vi "RSLT_VALUE.vi"(0 "MAX-MIN Temp":cluster{"MIN":dbl, "MAX":dbl, "ACTUAL":dbl}, 3 "INPUT cluster":T2, 5 "MAX-MIN PRESSURE":cluster{"MIN":dbl, "MAX":dbl, "ACTUALLY":dbl}, 7 "MAX-MIN FLOW":cluster{"MIN":dbl, "MAX":dbl, "ACTUALLY":dbl}, 9 "CLUSTER":T3={"Files"=[], "Browse File"=path "", "TIMEOUT"=100, "GRAPH"=[{array[68443 elements], array[68443 elements]}, {array[68363 elements], array[68363 elements]}, {array[40500 elements], array[40500 elements]}], "CHL 1"={"chl1 MIN"=110.0, "chl1 MAX"=130.0, "chl1 thrshold"=120.0}, "CHL 2"={"chl2 MIN"=33.0, "chl2 MAX"=35.0, "chl2 thrshold"=25.0}, "CHL 3"={"chl3 MIN"=20.0, "chl3 MAX"=30.0, "chl3 thrshold"=34.0}, "Report File"=path "", "Data_to_report"={"date/time string"="", "User Name"="", "BARCODE"="", "SELECTED RECIPE"="", "Rst"="", "Error Code"="", "RESULT ARRAY"=[]}, "BMP"={"chl3 MIN"=0.0, "chl3 MAX"=0.0, "chl3 thrshold"=0.0}}, 11 "error in":errorcluster, 12 "ACTUAL BPM":dbl=32134659.0 format="%#_13g") -> (4 "CLUSTER TO SQL":T1, 6 "RESULT ARRAY":string[](array[string]), 15 "error OUT":errorcluster)   [LabVIEW 2017]
panel:
  out "appended array":dbl[](array[numeric])
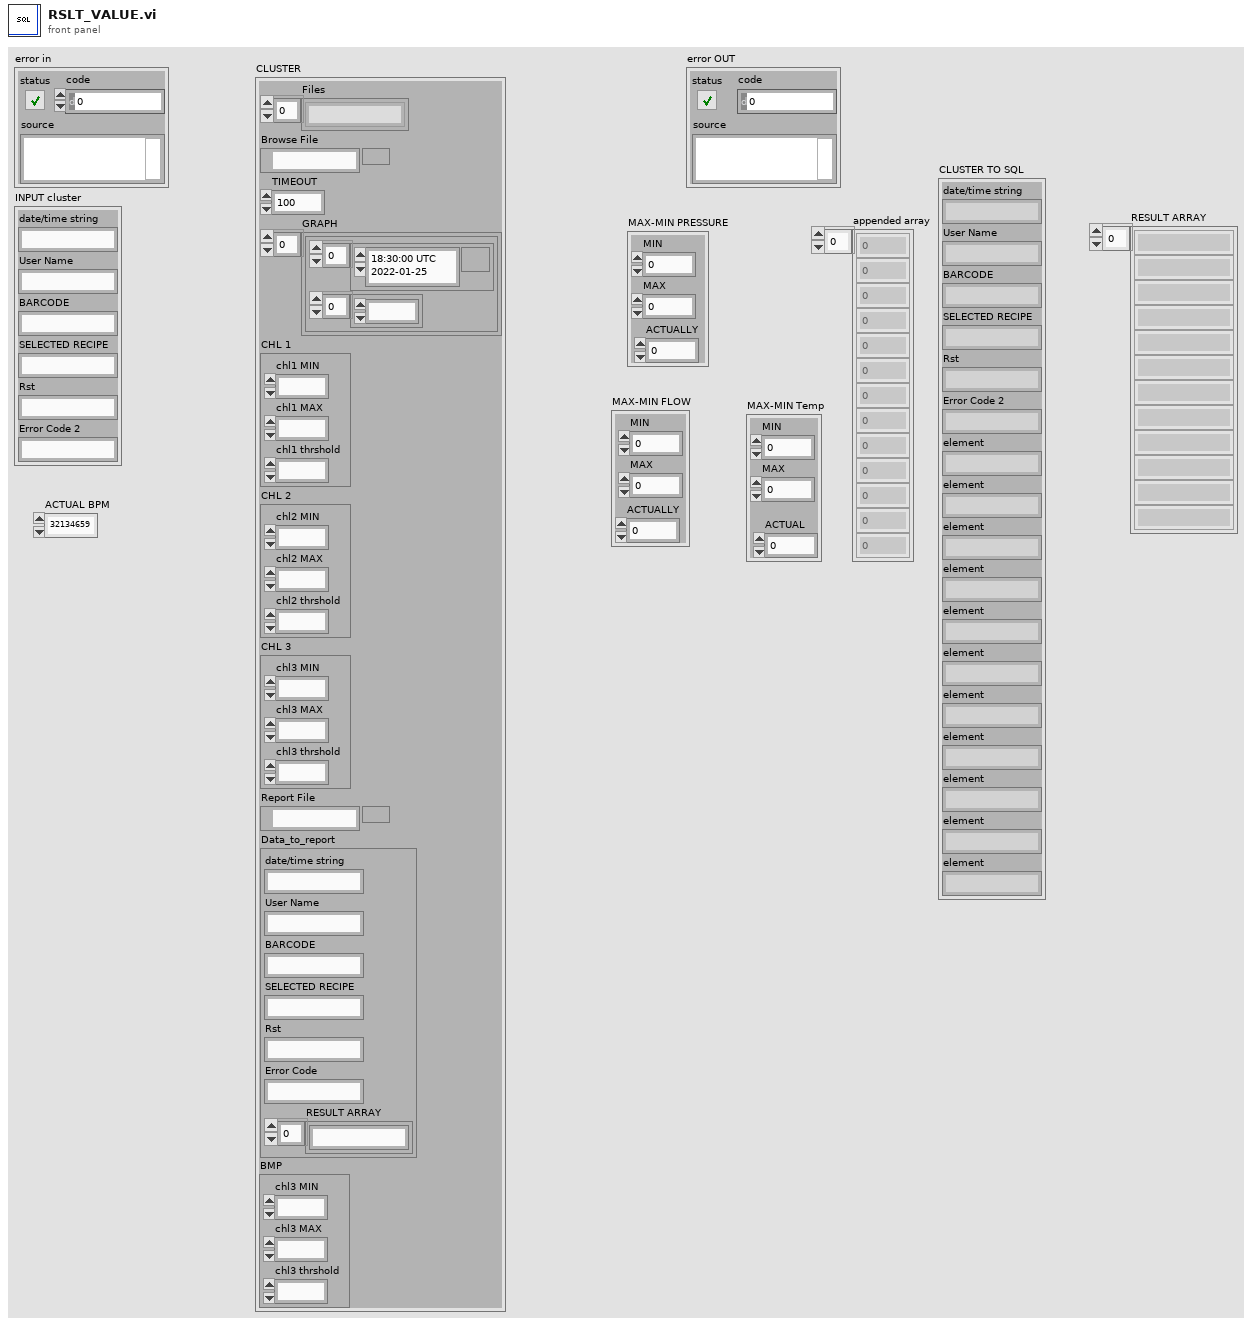
[diagram p1: front panel]
types:
  T1 = cluster{"date/time string":string, "User Name":string, "BARCODE":string, "SELECTED RECIPE":string, "Rst":string, "Error Code 2":string, "element":string, "element":string, "element":string, "element":string, "element":string, "element":string, "element":string, "element":string, "element":string, "element":string, "element":string}
  T2 = cluster{"date/time string":string, "User Name":string, "BARCODE":string, "SELECTED RECIPE":string, "Rst":string, "Error Code 2":string}
  T3 = cluster{"Files":string[], "Browse File":path, "TIMEOUT":i32, "GRAPH":cluster{timestamp[], ext[]}[], "CHL 1":cluster{"chl1 MIN":dbl, "chl1 MAX":dbl, "chl1 thrshold":dbl}, "CHL 2":cluster{"chl2 MIN":dbl, "chl2 MAX":dbl, "chl2 thrshold":dbl}, "CHL 3":cluster{"chl3 MIN":dbl, "chl3 MAX":dbl, "chl3 thrshold":dbl}, "Report File":path, "Data_to_report":cluster{"date/time string":string, "User Name":string, "BARCODE":string, "SELECTED RECIPE":string, "Rst":string, "Error Code":string, "RESULT ARRAY":string[]}, "BMP":cluster{"chl3 MIN":dbl, "chl3 MAX":dbl, "chl3 thrshold":dbl}}
  T4 = cluster{"date/time string":string, "User Name":string, "BARCODE":string, "SELECTED RECIPE":string, "Rst":string, "Error Code 2":string, "ACTUAL BPM":string, "ACTUAL BPM":string, "ACTUAL BPM":string, "ACTUAL BPM":string, "ACTUAL BPM":string, "ACTUAL BPM":string, "ACTUAL BPM":string, "ACTUAL BPM":string, "ACTUAL BPM":string, "ACTUAL BPM":string, "ACTUAL BPM":string}
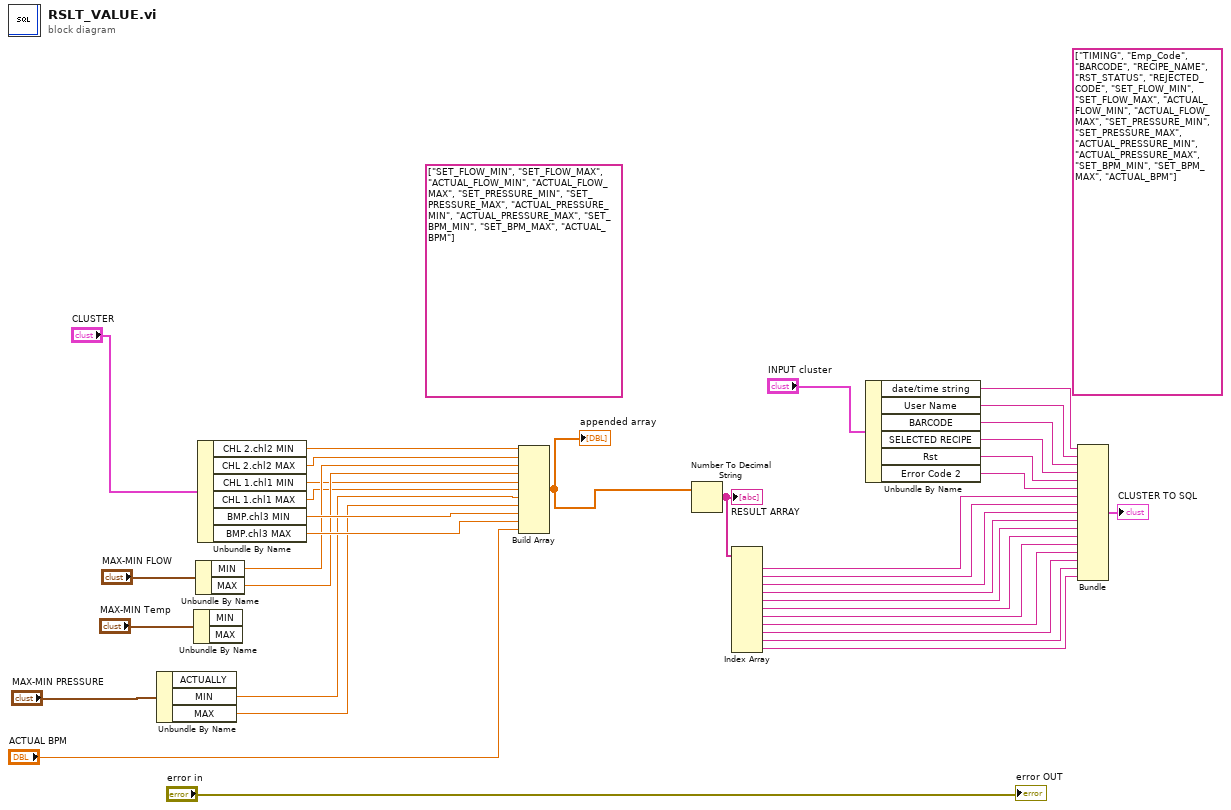
[diagram p0: block diagram]
diagram:
  (unwired) string[] ["TIMING", "Emp_Code", "BARCODE", "RECIPE_NAME", "RST_STATUS", "REJECTED_CODE", "SET_FLOW_MIN", "SET_FLOW_MAX", "ACTUAL_FLOW_MIN", "ACTUAL_FLOW_MAX", "SET_PRESSURE_MIN", "SET_PRESSURE_MAX", "ACTUAL_PRESSURE_MIN", "ACTUAL_PRESSURE_MAX", "SET_BPM_MIN", "SET_BPM_MAX", "ACTUAL_BPM"] ("columns")
  (unwired) string[] ["SET_FLOW_MIN", "SET_FLOW_MAX", "ACTUAL_FLOW_MIN", "ACTUAL_FLOW_MAX", "SET_PRESSURE_MIN", "SET_PRESSURE_MAX", "ACTUAL_PRESSURE_MIN", "ACTUAL_PRESSURE_MAX", "SET_BPM_MIN", "SET_BPM_MAX", "ACTUAL_BPM"] ("columns")
  n1 = Unbundle By Name("MAX-MIN PRESSURE") -> ("MIN"=w1:dbl, "MAX"=w2:dbl)  [unwired: 1 out]
  n2 = Unbundle By Name("MAX-MIN Temp") -> ()  [unwired: 2 out]
  n3 = Unbundle By Name("MAX-MIN FLOW") -> ("MIN"=w6:dbl, "MAX"=w5:dbl)
  n4 = Unbundle By Name("CLUSTER") -> ("CHL 2.chl2 MIN"=w34:dbl, "CHL 2.chl2 MAX"=w33:dbl, "CHL 1.chl1 MIN"=w4:dbl, "CHL 1.chl1 MAX"=w3:dbl, "BMP.chl3 MIN"=w32:dbl, "BMP.chl3 MAX"=w31:dbl)
  n5 = Build Array(w34, w33, w6, w5, w4, w3, w1, w2, w32, w31, "ACTUAL BPM") -> (w29:dbl[])
  "appended array" <- w29
  n6 = Number To Decimal String(number=w29) -> (decimal integer string=w26:string[])  [unwired: 1 in]
  "RESULT ARRAY" <- w26
  n7 = Index Array(array=w26) -> (element #1=w18:string, element #2=w17:string, element #3=w16:string, element #4=w15:string, element #5=w14:string, element #6=w13:string, element #7=w12:string, element #8=w11:string, element #9=w10:string, element #10=w9:string, element #11=w8:string)  [unwired: 11 in]
  n8 = Unbundle By Name("INPUT cluster") -> ("date/time string"=w24:string, "User Name"=w23:string, "BARCODE"=w22:string, "SELECTED RECIPE"=w21:string, "Rst"=w20:string, "Error Code 2"=w19:string)
  n9 = Bundle("date/time string"=w24, "User Name"=w23, "BARCODE"=w22, "SELECTED RECIPE"=w21, "Rst"=w20, "Error Code 2"=w19, "ACTUAL BPM"=w18, "ACTUAL BPM"=w17, "ACTUAL BPM"=w16, "ACTUAL BPM"=w15, "ACTUAL BPM"=w14, "ACTUAL BPM"=w13, "ACTUAL BPM"=w12, "ACTUAL BPM"=w11, "ACTUAL BPM"=w10, "ACTUAL BPM"=w9, "ACTUAL BPM"=w8) -> (→"CLUSTER TO SQL":T4)  [unwired: 1 in]
  "error OUT" <- "error in"
